vi "London.vi"() -> ()   [LabVIEW 2020]
panel:
  out "n CGS":dbl
  out "n":ext
  in  "London":dbl=2.2e-08 format="%#_6pm"
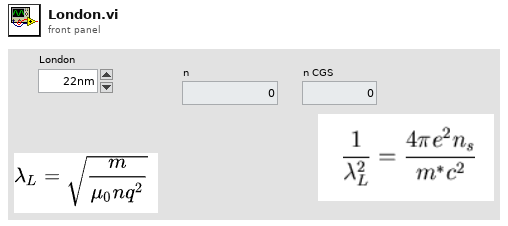
[diagram p1: front panel]
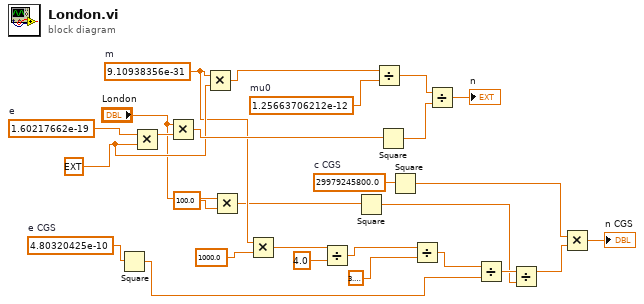
[diagram p0: block diagram]
diagram:
  w7 = 29979245800.0  # c CGS
  w9 = 4.80320425e-10  # e CGS
  w20 = 1.60217662e-19  # e
  w22 = ext 2.0 ("y")
  w27 = 1.25663706212e-12  # mu0
  w16 = 9.10938356e-31  # m
  n1 = Square(x=w9) -> (x^2=w1:dbl)
  n2 = Multiply(x=w20, y=w22) -> (x*y=w23:ext)
  n3 = Multiply(x="London", y=w23) -> (x*y=w26:ext)
  n4 = Multiply(x=w16, y=w22) -> (x*y=w21:ext)
  n5 = Multiply(x="London", y=100.0) -> (x*y=w3:dbl)
  n6 = Multiply(x=w16, y=1000.0) -> (x*y=w14:dbl)
  n7 = Divide(x=w14, y=4.0) -> (x/y=w12:dbl)
  n8 = Square(x=w3) -> (x^2=w2:dbl)
  n9 = Divide(x=w21, y=w27) -> (x/y=w24:ext)
  n10 = Square(x=w26) -> (x^2=w25:ext)
  n11 = Square(x=w7) -> (x^2=w6:dbl)
  n12 = Divide(x=w12, y=3.141592653589793) -> (x/y=w10:dbl)
  n13 = Divide(x=w24, y=w25) -> (x/y=→"n":ext)
  n14 = Divide(x=w10, y=w1) -> (x/y=w8:dbl)
  n15 = Divide(x=w8, y=w2) -> (x/y=w4:dbl)
  n16 = Multiply(x=w6, y=w4) -> (x*y=→"n CGS":dbl)
